vi "Compile Component.vi"(9 "Options (Default)":T2, 10 "Encoding Callback":refnum<vi>, 11 "Input":string) -> (0 "error IO":errorcluster, 3 "Component":T1)   [LabVIEW 2020, in "Stream.lvlib" / "URLPattern.lvclass"]
uses:
  URLPattern.lvclass
  Pattern String Options.ctl
  Component.ctl
  RegExp Flags.ctl
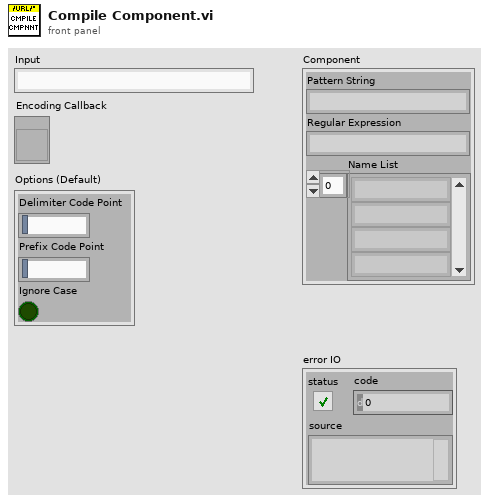
[diagram p1: front panel]
types:
  T1 = typedef "Stream.lvlib/URLPattern.lvclass/Component.ctl" = cluster{"Pattern String":string, "Regular Expression":string, "Name List":string[]}
  T2 = typedef "Stream.lvlib/URLPattern.lvclass/Pattern String Options.ctl" = cluster{"Delimiter Code Point":string, "Prefix Code Point":string, "Ignore Case":bool}
  T3 = typedef "Stream.lvlib/URLPattern.lvclass/Pattern Part.ctl" = cluster{"Type":T4, "Value":string, "Modifier":T5, "Name":string, "Prefix":string, "Suffix":string}
  T4 = typedef "Stream.lvlib/URLPattern.lvclass/Pattern Part Type.ctl" = enum16{"fixed-text", "regexp", "segment-wildcard", "full-wildcard"}
  T5 = typedef "Stream.lvlib/URLPattern.lvclass/Pattern Part Modifier.ctl" = enum16{"none", "optional", "zero-or-more", "one-or-more"}
  T6 = typedef "Stream.lvlib/URLPattern.lvclass/RegExp Flags.ctl" = cluster{"Ignore Case":bool, "Multiline":bool}
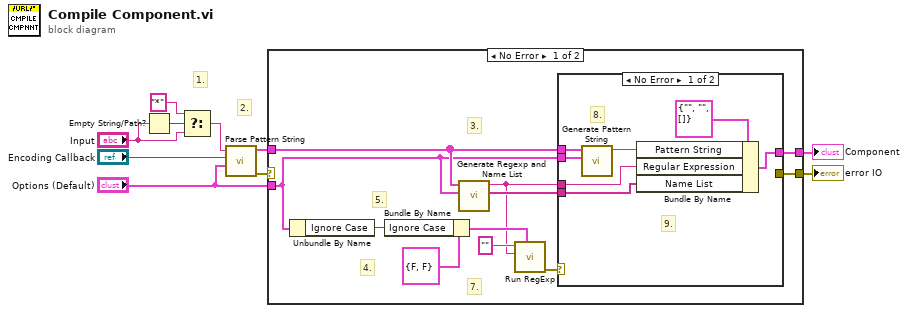
[diagram p0: block diagram]
diagram:
  # "2."
  # "1."
  n1 = Empty String/Path?(string/path="Input") -> (empty?=w10:bool)
  n2 = Select(t="*", s=w10, f="Input") -> (s? t:f=w7:string)
  n3 = call "Parse Pattern String.vi"("Options (Default)"="Options (Default)", "Encoding Callback"="Encoding Callback", "Input"=w7) -> ("error out"=w5:errorcluster, "Part List"=w4:T3[])  [unwired: 7 in]
  n4 = case shown="No Error" w5 {
    selector: w5 -> [_ w30]
    tunnel: w4 -> [w15 _]
    tunnel: "Options (Default)" -> [w11 _]
    tunnel: [w16 w30] -> w1
    tunnel: [w12 _] -> w2
    frame No Error {
      # "7."
      # "5."
      # "4."
      # "3."
      n5 = Unbundle By Name(w11) -> ("Ignore Case"=w20:bool)
      n6 = Bundle By Name(cluster=T6 {"Ignore Case"=FALSE, "Multiline"=FALSE} ("RegExp Flags"), "Ignore Case"=w20) -> (w19:T6)
      n7 = call "Generate Regexp and Name List.vi"("Options (Default)"=w11, "Part List"=w15) -> ("Name List"=w14:string[], "Result"=w13:string)  [unwired: 8 in]
      n8 = call "Run RegExp.vi"("flags"=w19, "regular expression"=w13, "string"="") -> ("error out"=w18:errorcluster)  [unwired: 4 in, 4 out]
      n9 = case shown="No Error" w18 {
        selector: w18 -> [_ w29]
        tunnel: [_ w29] -> w16
        tunnel: w15 -> [w28 _]
        tunnel: w11 -> [w27 _]
        tunnel: w14 -> [w23 _]
        tunnel: w13 -> [w24 _]
        tunnel: [w22 _] -> w12
        frame No Error {
          # "9."
          # "8."
          n10 = call "Generate Pattern String.vi"("Options (Default)"=w27, "Part List"=w28) -> ("Result"=w25:string)  [unwired: 9 in]
          n11 = Bundle By Name(cluster=T1 {"Pattern String"="", "Regular Expression"="", "Name List"=[]} ("Component"), "Pattern String"=w25, "Regular Expression"=w24, "Name List"=w23) -> (w22:T1)
        }
        frame Error {
        }
      }
    }
    frame Error {
    }
  }
  "Component" <- w2
  "error IO" <- w1
